vi "Remove JSON Tag.vi"(11 "Name":string) -> (2 "Tag":T1, 3 "Name (tag stripped)":string)   [LabVIEW 2020, in "JSONtext.lvlib"]
uses:
  <vilib>/JDP Science/JSONtext/JSONtext.lvlib
  <vilib>/JDP Science/JSONtext/support/Tag Type.ctl
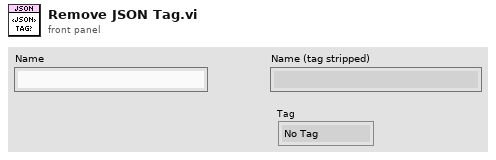
[diagram p1: front panel]
types:
  T1 = typedef "JSONtext.lvlib/Tag Type.ctl" = enum16{"No Tag", "<JSON>", "<JOBJ>"}
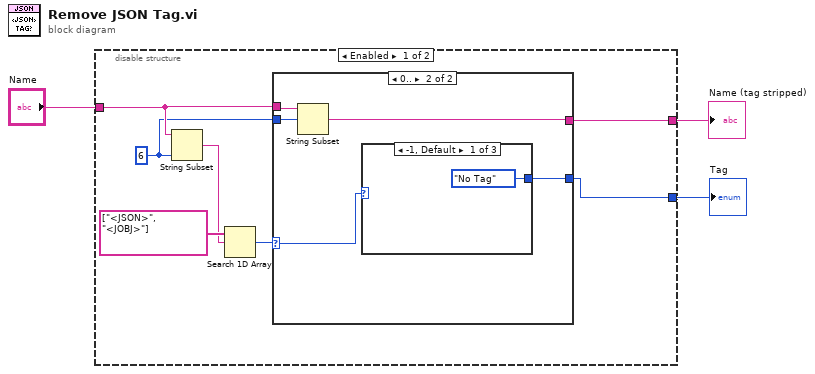
[diagram p0: block diagram]
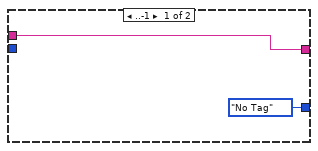
[diagram p2: hidden frame]
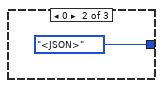
[diagram p3: hidden frame]
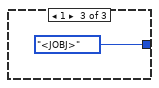
[diagram p4: hidden frame]
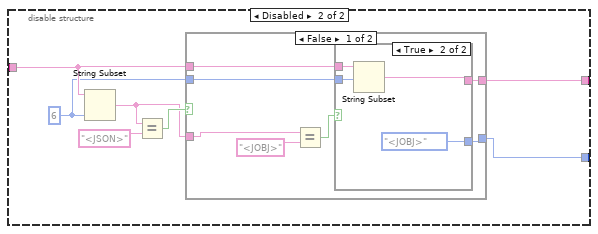
[diagram p5: hidden frame]
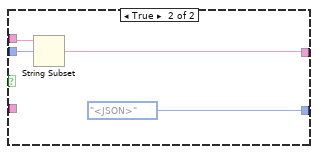
[diagram p7: hidden frame]
diagram:
  n1 = disable-structure shown="Enabled" {
    disable-tunnel: "Name" -> [w10 w26]
    disable-tunnel: [w9 w25] -> w2
    disable-tunnel: [w7 w21] -> w1
    frame Enabled {
      w8 = 6 ("length (rest)")
      n2 = String Subset(string=w10, length (rest)=w8) -> (substring=w5:string)  [unwired: 1 in]
      n3 = Search 1D Array(1D array=string[] ["<JSON>", "<JOBJ>"], element=w5) -> (index of element=w4:i32)  [unwired: 1 in]
      n4 = case shown="0.." w4 {
        selector: w4 -> [_ w14]
        tunnel: [w12 w16] -> w9
        tunnel: w10 -> [w12 w17]
        tunnel: w8 -> [_ w13]
        tunnel: [Tag_Type."No Tag" ("Tag") w15] -> w7
        frame ..-1 {
        }
        frame 0.. {
          n5 = String Subset(string=w17, offset (0)=w13) -> (substring=w16:string)  [unwired: 1 in]
          n6 = case shown="-1, Default" w14 {
            tunnel: [Tag_Type."No Tag" ("Tag") Tag_Type."<JSON>" ("Tag") Tag_Type."<JOBJ>" ("Tag")] -> w15
            frame -1, Default {
            }
            frame 0 {
            }
            frame 1 {
            }
          }
        }
      }
    }
    frame Disabled {
      w23 = 6 ("length (rest)")
      n7 = String Subset(string=w26, length (rest)=w23) -> (substring=w22:string)  [unwired: 1 in]
      n8 = Equal?(x=w22, y="<JSON>") -> (x = y?=w27:bool)
      n9 = case shown="False" w27 {
        tunnel: [w31 w42] -> w25
        tunnel: w26 -> [w32 w43]
        tunnel: w23 -> [w30 w41]
        tunnel: w22 -> [w33 _]
        tunnel: [w28 Tag_Type."<JSON>" ("Tag")] -> w21
        frame False {
          n10 = Equal?(x=w33, y="<JOBJ>") -> (x = y?=w29:bool)
          n11 = case shown="True" w29 {
            tunnel: w32 -> [w35 w39]
            tunnel: [w35 w38] -> w31
            tunnel: w30 -> [_ w37]
            tunnel: [_ Tag_Type."<JOBJ>" ("Tag")] -> w28
            frame False {
            }
            frame True {
              n12 = String Subset(string=w39, offset (0)=w37) -> (substring=w38:string)  [unwired: 1 in]
            }
          }
        }
        frame True {
          n13 = String Subset(string=w43, offset (0)=w41) -> (substring=w42:string)  [unwired: 1 in]
        }
      }
    }
  }
  "Tag" <- w1
  "Name (tag stripped)" <- w2
